vi "Connection State Callback.vi"(7 "Owner":refnum<class>, 10 "Connection State":T1, 11 "Endpoint":refnum<class "Endpoint.lvclass">) -> ()   [LabVIEW 2020, in "LV Client.lvclass"]
uses:
  LV Client.lvclass
  LV Client.lvclass/LV Client.ctl
  <vilib>/IlluminatedG/lv-stream/Connection State.ctl
  <vilib>/IlluminatedG/lv-stream/Stream.lvlib
  <vilib>/IlluminatedG/lv-msg-simple/Stream-Simple-Msg/Endpoint/Endpoint.lvclass
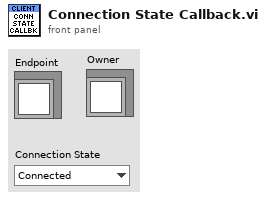
[diagram p1: front panel]
types:
  T1 = typedef "Stream.lvlib/Connection State.ctl" = enum16{"Connected", "Disconnected"}
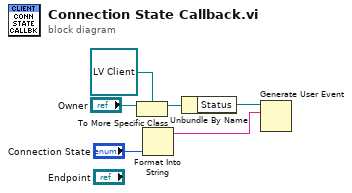
[diagram p0: block diagram]
diagram:
  n1 = To More Specific Class(target class=refnum<class "LV Client.lvclass"> refnum ("LV Client.lvclass"), reference="Owner") -> (specific class reference=w3:refnum<class "LV Client.lvclass">)  [unwired: 1 in, 1 out]
  n2 = Format Into String("Connection State") -> (resulting string=w1:string)  [unwired: 3 in, 1 out]
  n3 = Unbundle By Name(w3) -> ("Status"=w2:refnum<user-event>)
  n4 = Generate User Event(user event=w2, event data cluster=w1) -> ()  [unwired: 2 in, 2 out]
